vi "data string match.vi"() -> ()   [LabVIEW 2014]
panel:
  in  "Array":dbl[](array[numeric])
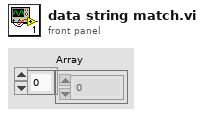
[diagram p1: front panel]
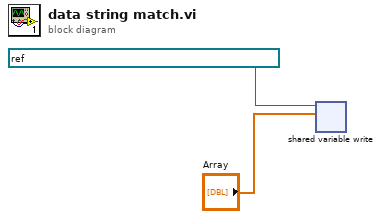
[diagram p0: block diagram]
diagram:
  n1 = shared-variable-write(refnum<k21> "ni.var.psp://my computer/Test Data/testdata1" ("shared variable refnum in"), "Array") -> ()  [unwired: 1 in, 2 out]
